vi "_API_BINANCE_GET_SymbolOrderBookTicker.vi"(0 "BinanceAPI in":refnum<class "BinanceAPI_.lvclass">, 5 "SymbolOrderBookTicker":cluster{"symbol":string}, 11 "error in (no error)":errorcluster) -> (4 "BinanceAPI out":refnum<class "BinanceAPI_.lvclass">, 6 "Data":T1, 14 "Data":string, 15 "error out":errorcluster)   [LabVIEW 2022 SP3, in "BinanceAPI_.lvclass"]
doc: "https://binance-docs.github.io/apidocs/spot/en/#symbol-order-book-ticker"
uses:
  BinanceAPI_.lvclass
  BinanceAPI_.lvclass/BinanceAPI_.ctl
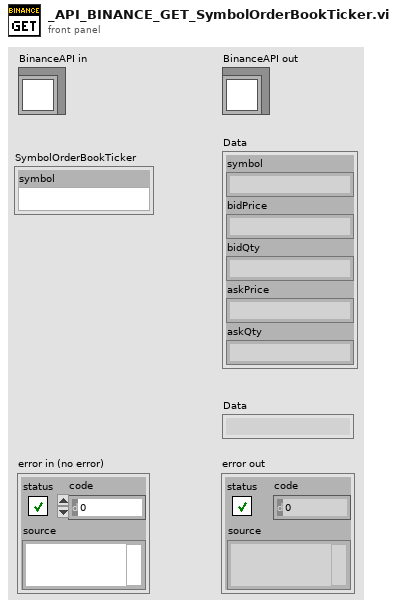
[diagram p1: front panel]
types:
  T1 = cluster{"symbol":string, "bidPrice":string, "bidQty":string, "askPrice":string, "askQty":string}
  T2 = typedef "LabVIEWHTTPClient.lvlib/ClientHandle.ctl" = refnum<k1>
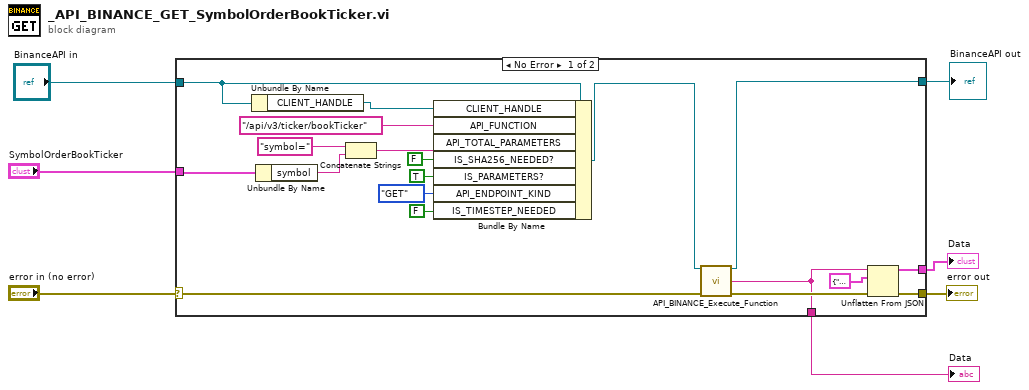
[diagram p0: block diagram]
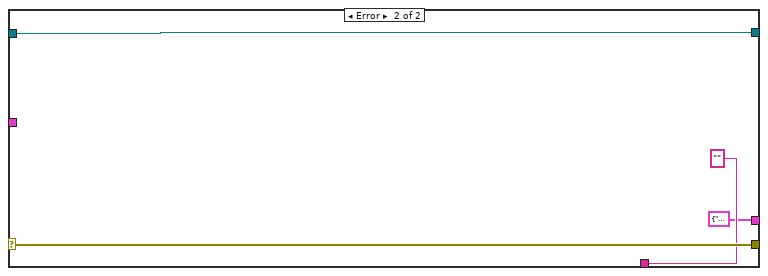
[diagram p2: hidden frame]
diagram:
  n1 = case shown="No Error" "error in (no error)" {
    selector: "error in (no error)" -> [w14 w30]
    tunnel: [w11 w30] -> w6
    tunnel: [w15 w29] -> w1
    tunnel: "BinanceAPI in" -> [w23 w29]
    tunnel: "SymbolOrderBookTicker" -> [w19 _]
    tunnel: [w10 "" ("Dane")] -> w4
    tunnel: [w8 T1 {"symbol"="", "bidPrice"="", "bidQty"="", "askPrice"="", "askQty"=""}] -> w3
    frame No Error {
      n2 = Unbundle By Name(w23) -> ("CLIENT_HANDLE"=w24:T2)
      n3 = Unbundle By Name(w19) -> ("symbol"=w21:string)
      n4 = Concatenate Strings("symbol=" ("API_FUNCTION 2"), w21) -> (w20:string)
      n5 = Bundle By Name(cluster=w23, "CLIENT_HANDLE"=w24, "API_FUNCTION"="/api/v3/ticker/bookTicker", "API_TOTAL_PARAMETERS"=w20, "IS_SHA256_NEEDED?"=FALSE, "IS_PARAMETERS?"=TRUE, "API_ENDPOINT_KIND"=enum16{"POST", "DELETE", "GET", "PUT"}."GET", "IS_TIMESTEP_NEEDED"=FALSE) -> (w16:refnum<class "BinanceAPI_.lvclass">)
      n6 = call "API_BINANCE_Execute_Function.vi"("BinanceAPI in"=w16, "error in (no error)"=w14) -> ("BinanceAPI out"=w15:refnum<class "BinanceAPI_.lvclass">, "Body"=w10:string, "error out"=w12:errorcluster)  [unwired: 9 in, 2 out]
      n7 = Unflatten From JSON(JSON string=w10, type and defaults=T1 {"symbol"="", "bidPrice"="", "bidQty"="", "askPrice"="", "askQty"=""}, error in (no error)=w12) -> (value=w8:T1, error out=w11:errorcluster)  [unwired: 4 in]
    }
    frame Error {
    }
  }
  "error out" <- w6
  "Data" <- w4
  "Data" <- w3
  "BinanceAPI out" <- w1
